vi "Save Profile.vi"(9 "Profile":string[][](array[string]), 10 "Current Profile":string, 11 "Profiles Path":path) -> (3 "Profile OUT":string[][](array[string]))   [LabVIEW 2019]
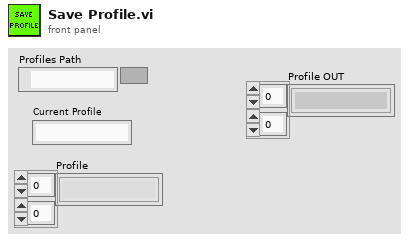
[diagram p1: front panel]
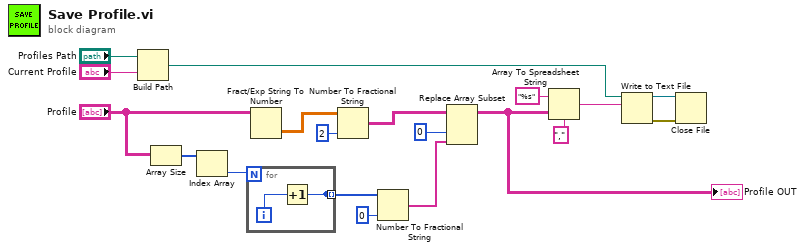
[diagram p0: block diagram]
diagram:
  n1 = Build Path(base path="Profiles Path", name or relative path="Current Profile") -> (appended path=w19:path)
  n2 = Array Size(array="Profile") -> (size(s)=w12:i32[])
  n3 = Index Array(array=w12) -> (element=w11:i32)  [unwired: 1 in]
  n4 = for {
    N: w11 -> [_]
    tunnel: [w20] -> _ mode=indexing
    tunnel: [w20] -> w10 mode=indexing
    i -> [w21]
    n5 = Increment(x=w21) -> (x+1=w20:i32)
  }
  n6 = Fract/Exp String To Number(string="Profile") -> (number=w3:dbl[][])  [unwired: 3 in, 1 out]
  n7 = Number To Fractional String(number=w3, precision (6)=i16 2) -> (F-format string=w1:string[][])  [unwired: 2 in]
  n8 = Number To Fractional String(number=w10, precision (6)=i16 0) -> (F-format string=w8:string[])  [unwired: 2 in]
  n9 = Replace Array Subset(array=w1, new element=w8, index (col)=0 ("disabled index (col)")) -> (w5:string[][])  [unwired: 1 in]
  "Profile OUT" <- w5
  n10 = Array To Spreadsheet String(delimiter (Tab)=",", array=w5, 3:"%s" ("format string")) -> (spreadsheet string=w6:string)
  n11 = Write to Text File(file (use dialog)=w19, text=w6) -> (refnum out=w18:refnum<file>, error out=w17:errorcluster)  [unwired: 2 in, 1 out]
  n12 = Close File(refnum=w18, error in=w17) -> ()  [unwired: 2 out]
